vi "cse360_temp_logger.vi"() -> ()   [LabVIEW 2020]
uses:
  <vilib>/Instr/_visa.llb/VISA Configure Serial Port (Instr).vi
panel:
  out "Instructions":string
  in  "Off / On":bool
  in  "file path (use dialog)":path
  out "path":path
  out "error out":errorcluster
  out "Temp Chart":dbl(graph)
  in  "Select com port":refnum<visa-resource-name>
  out "celsius (c)":dbl
  out "Thermometer":dbl(slide) scale=0.0..100.0
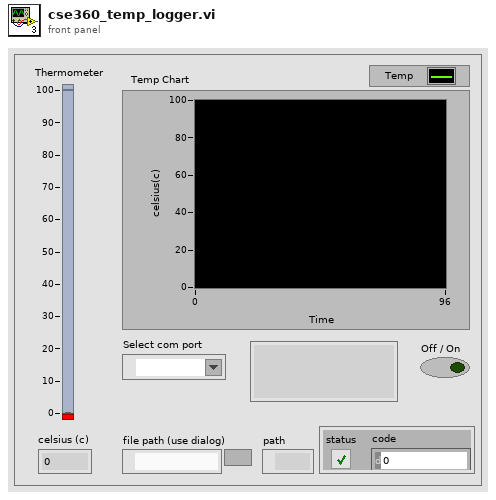
[diagram p1: front panel]
types:
  T1 = enum16{"open", "replace", "create", "open or create", "replace or create", "replace or create with confirmation"}
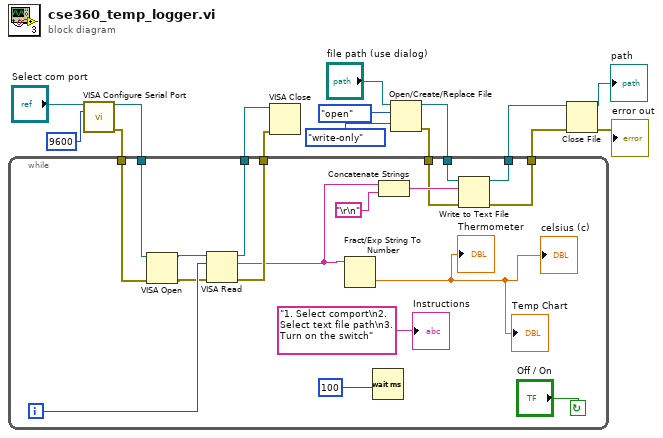
[diagram p0: block diagram]
diagram:
  n1 = call-poly "VISA Configure Serial Port"("VISA resource name"="Select com port", "baud rate (9600)"=u32 9600) -> ("VISA resource name out"=w4:refnum<visa-resource-name>, "error out"=w3:errorcluster)  [unwired: 12 in]
  n2 = Open/Create/Replace File(file path (use dialog)="file path (use dialog)", operation (0:open)=T1."open", access (0:read/write)=enum16{"read/write", "read-only", "write-only"}."write-only") -> (refnum out=w2:refnum<file>, error out=w1:errorcluster)  [unwired: 3 in, 1 out]
  n3 = while {
    tunnel: [w33] -> w13
    tunnel: [w32] -> w12
    tunnel: [w23] -> w7
    tunnel: [w22] -> w6
    tunnel: w4 -> [w21]
    tunnel: w3 -> [w20]
    tunnel: w2 -> [w19]
    tunnel: w1 -> [w18]
    i -> [w31]
    stop <- "Off / On" continue-if-true
    n4 = VISA Open(error in (no error)=w20, VISA resource name=w21) -> (VISA resource name=w30:refnum<visa-resource-name>, error out=w29:errorcluster)  [unwired: 3 in]
    n5 = VISA Read(VISA resource name=w30, byte count=w31, error in (no error)=w29) -> (VISA resource name out=w33:refnum<visa-resource-name>, read buffer=w26:string, error out=w32:errorcluster)  [unwired: 1 out]
    n6 = Fract/Exp String To Number(string=w26) -> (number=→"Thermometer" →"celsius (c)" →"Temp Chart":dbl)  [unwired: 3 in, 1 out]
    n7 = Wait (ms)(milliseconds to wait=u32 100 ("baud rate (9600)")) -> ()  [unwired: 1 out]
    n8 = Concatenate Strings(w26, "\r\n") -> (w24:string)
    n9 = Write to Text File(file (use dialog)=w19, text=w24, error in=w18) -> (refnum out=w23:refnum<file>, error out=w22:errorcluster)  [unwired: 1 in, 1 out]
    "Instructions" <- "1. Select comport\n2. Select text file path\n3. Turn on the switch"
  }
  n10 = VISA Close(VISA resource name=w13, error in (no error)=w12) -> ()  [unwired: 1 out]
  n11 = Close File(refnum=w7, error in=w6) -> (path=→"path":path, error out=→"error out":errorcluster)
